vi "Begin.vi"(8 "error in":errorcluster) -> (0 "error out":errorcluster)   [LabVIEW 2015]
doc: "Called before other user functions, this VI is expected to open initial I/O refnums, load in file data, and do all program initialization. Notice that the <B>error out</B> terminal is simply used for data flow. Wiring it to other structures or subVIs ensures that this VI runs first."
uses:
  <vilib>/Rock Robotics/SystemInterfaces/i2clib/i2c_bus.ctl
  <vilib>/Rock Robotics/WPI/DriverStation/WPI_DriverStationRobotMode2.ctl
  <vilib>/Rock Robotics/SystemInterfaces/DIO/FPGA_DIOPWMChannel.ctl
  <vilib>/Rock Robotics/SystemInterfaces/spilib/spi_bus.ctl
  <vilib>/Rock Robotics/WPI/Accelerometer/WPI_AccelerometerADXL345 Axes.ctl
  <vilib>/Rock Robotics/WPI/Accelerometer/ADXL362 Range.ctl
  Robot Global Data.vi
  <vilib>/Rock Robotics/Network Tables/NT Write String Array.vi
  Team Code/Global_Var/Drive_Global.vi
  <vilib>/Rock Robotics/WPI/Gyro/WPI_GyroXRS450_SPI_Open.vi
  <vilib>/Rock Robotics/WPI/Accelerometer/WPI_AccelerometerADXL362_SPI_Open.vi
panel:
  in  "Comp_Robot?":bool=TRUE
  out "IMU Cal Result":T1={"AccelCalGood"=FALSE, "GyroCalGood"=TRUE, "MagCalGood"=FALSE, "Accel_StdDev"=0.2675184573071548, "Gyro_StdDev"=0.04462048242979951}
  in  "NumCalSamples":i32=50
  in  "Accel-Gyro_Settings":T2={"Accel_Range"=enum."±4g", "Gyro_Range"=enum."±500dps", "A/G_Address"=enum."0x6B", "Motion Thresh"=0.0, "reset"=FALSE}
  in  "Mag_Settings":T3={"Mag_Range"=enum."±2 gauss", "Mag_Address"=enum."0x1E", "Anomaly Thresh"=0.0, "Local Mag"=0.0}
  in  "I2C Bus":T4
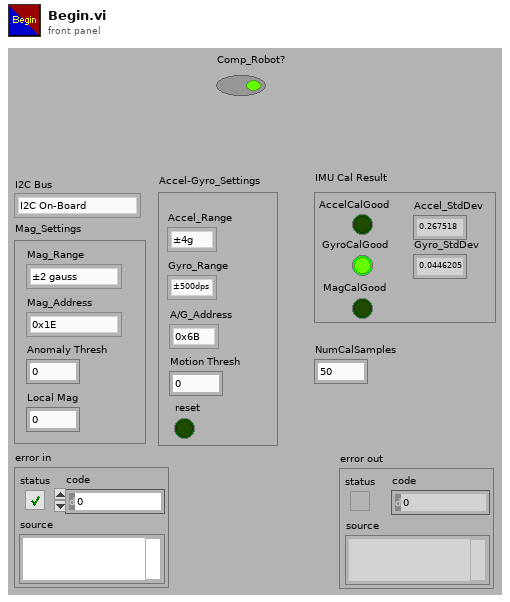
[diagram p1: front panel]
types:
  T1 = cluster{"AccelCalGood":bool, "GyroCalGood":bool, "MagCalGood":bool, "Accel_StdDev":dbl, "Gyro_StdDev":dbl}
  T2 = cluster{"Accel_Range":enum8{"±2g", "±16g", "±4g", "±8g", "disabled"}, "Gyro_Range":enum8{"±245dps", "±500dps", "disabled", "±2000dps"}, "A/G_Address":enum8{"0x6A", "0x6B"}, "Motion Thresh":dbl, "reset":bool}
  T3 = cluster{"Mag_Range":enum8{"±2 gauss", "±4 gauss", "±8 gauss", "±16 gauss", "disabled"}, "Mag_Address":enum8{"0x1C", "0x1E"}, "Anomaly Thresh":dbl, "Local Mag":dbl}
  T4 = typedef "i2c_bus.ctl" = enum16{"I2C On-Board", "I2C MXP", "Invalid"}
  T5 = typedef "ADXL362 Range.ctl" = u8
  T6 = typedef "WPI_AccelerometerADXL345 Axes.ctl" = cluster{"X-Axis":bool, "Y-Axis":bool, "Z-Axis":bool}
  T7 = typedef "spi_bus.ctl" = enum16{"SPI On-Board, CS0", "SPI On-Board, CS1", "SPI On-Board, CS2", "SPI On-Board, CS3", "SPI MXP", "Invalid"}
  T8 = typedef "FPGA_DIOPWMChannel.ctl" = enum8{"PWM 0", "PWM 1", "PWM 2", "PWM 3", "PWM 4", "PWM 5", "PWM 6", "PWM 7", "PWM 8", "PWM 9", "PWM MXP 0", "PWM MXP 1", "PWM MXP 2", "PWM MXP 3", "PWM MXP 4", "PWM MXP 5", "PWM MXP 6", "PWM MXP 7", "PWM MXP 8", "PWM MXP 9", "Invalid"}
  T9 = typedef "WPI_DriverStationRobotMode2.ctl" = enum16{"Autonomous Disabled", "Autonomous Enabled", "Teleop Disabled", "Teleop Enabled", "Disconnected", "Finish", "Test Disabled", "Test Enabled", "Emergency Stopped"}
  T10 = typedef "LSM9DS1DevRef.ctl" = cluster{"DevStatus":errorcluster, "Gyro Offset":cluster{"Xzero":dbl, "Yzero":dbl, "Zzero":dbl}, "StdDev Rates":cluster{"Xsdo":dbl, "Ysdo":dbl, "Zsdo":dbl}, "Reset":bool, "Accel Offset":cluster{"Xzero":dbl, "Yzero":dbl, "Zzero":dbl}, "Motion Thresh":dbl, "Mag Offset":cluster{"Xzero":dbl, "Yzero":dbl, "Zzero":dbl}, "I2C Bus":T4, "Handle":i32, "Anomaly Thresh":dbl, "Local Mag":dbl, "Accel/Gyro_Address":enum8{"0x6A", "0x6B"}, "Accel_Range":enum16{"±2g", "±16g", "±4g", "±8g", "disabled"}, "Gyro_Range":enum16{"±245dps", "±500dps", "disabled", "±2000dps"}, "Mag_Range":enum16{"±2 gauss", "±4 gauss", "±8 gauss", "±16 gauss", "disabled"}, "Mag_Address":enum8{"0x1C", "0x1E"}, "accel_active":bool, "gyro_active":bool, "mag_active":bool}
  T11 = typedef "WPI_ServoDeviceRef.ctl" = cluster{"DeviceStatus":errorcluster, "PWM Channel":T8, "DeadBand":T12}
  T12 = typedef "WPI_PWMDeadband.ctl" = cluster{"Name":string, "maxPositivePwm":i32, "minPositivePwm":i32, "centerPwm":i32, "maxNegativePwm":i32, "minNegativePwm":i32, "angularRange":u16}
  T13 = typedef "WPI_GyroDevRef.ctl" = cluster{"DevStatus":errorcluster, "Analog Channel":T14, "Offset":dbl, "Gain (VoltsPerDegree/Second)":dbl, "Gyro Type":enum16{"Analog", "XRS450"}, "Handle":i32, "SPI Bus":T7, "Device Found":bool, "Sample Rate":dbl, "Calibrate On Open":bool}
  T14 = typedef "FPGA_AIChannel.ctl" = enum8{"AI 0", "AI 1", "AI 2", "AI 3", "AI MXP 0", "AI MXP 1", "AI MXP 2", "AI MXP 3", "Invalid"}
  T15 = typedef "WPI_AccelerometerDevRef.ctl" = cluster{"DevStatus":errorcluster, "Scaling":T16, "Analog Channels":T17, "I2C Bus":T4, "SPI Bus":T7, "Accel Range":T18, "ADXL Axes":T6, "Handle":i32, "Device Address":u8, "Accel Type":enum16{"Analog", "ADXL345 I2C", "ADXL345 SPI", "Internal", "ADXL362 SPI"}}
  T16 = typedef "WPI_AccelerometerScaling.ctl" = cluster{"Gain (VoltsPerG)":dbl, "Center Voltage":dbl}
  T17 = typedef "WPI_AccelerometerAnalogChannels.ctl" = cluster{"X-Axis":T14, "Y-Axis":T14, "Z-Axis":T14}
  T18 = typedef "ADXL345 Range.ctl" = u8
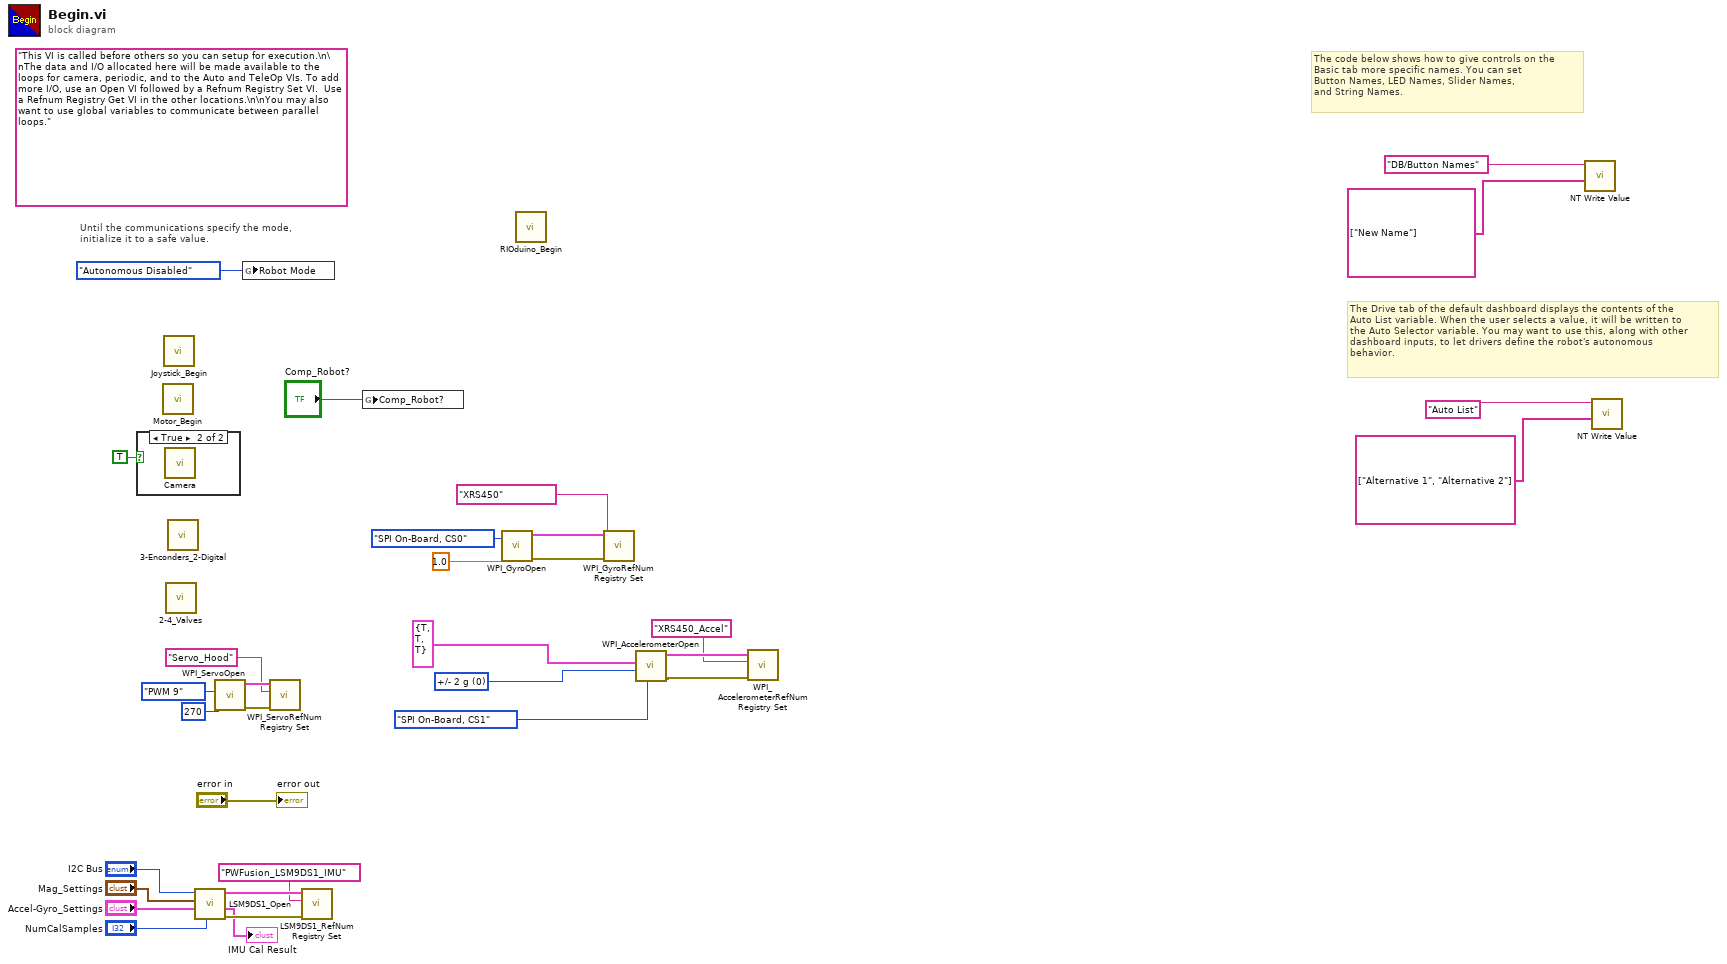
[diagram p0: block diagram]
diagram:
  w5 = T5 0 items=["+/- 2 g", "+/- 4 g", "+/- 8 g"] ("Accel Range")
  (unwired) "This VI is called before others so you can setup for execution.\n\nThe data and I/O allocated here will be made available to the loops for camera, periodic, and to the Auto and TeleOp VIs. To add more I/O, use an Open VI followed by a Refnum Registry Set VI.  Use a Refnum Registry Get VI in the other locations.\n\nYou may also want to use global variables to communicate between parallel loops."
  # "The Drive tab of the default dashboard displays the contents of the\nAuto List variable. When the user selects a value, it will be written to\nthe Auto Selector variable. You may want to use this, along with other\ndashboard inputs, to let drivers define the robot's autonomous\nbehavior."
  # "The code below shows how to give controls on the\nBasic tab more specific names. You can set\nButton Names, LED Names, Slider Names,\nand String Names."
  # "Until the communications specify the mode,\ninitialize it to a safe value."
  n1 = case shown="True" TRUE {
    frame False {
    }
    frame True {
      n2 = call "Camera.vi"() -> ()  [unwired: 12 in]
    }
  }
  n3 = call "Motor_Begin.vi"() -> ()  [unwired: 12 in]
  n4 = call "Joystick_Begin.vi"() -> ()  [unwired: 12 in]
  n5 = call "2-4_Valves.vi"() -> ()  [unwired: 12 in]
  n6 = call "3-Enconders_2-Digital.vi"() -> ()  [unwired: 12 in]
  n7 = call "LSM9DS1_Open.vi"("NumCalSamples"="NumCalSamples", "Accel-Gyro_Settings"="Accel-Gyro_Settings", "Mag_Settings"="Mag_Settings", "I2C Bus"="I2C Bus") -> ("error out"=w23:errorcluster, "IMU Cal Result"=→"IMU Cal Result":T1, "LSM9DS1DevRef Out"=w25:T10)  [unwired: 5 in]
  n8 = call <vilib>:"WPI_ServoOpen.vi"("Angular Range"=u16 270, "PWM Channel"=FPGA_DIOPWMChannel."PWM 9") -> ("error out"=w16:errorcluster, "ServoDeviceRef"=w15:T11)  [unwired: 8 in]
  n9 = global write "Robot Global Data.vi" "Robot Mode"(WPI_DriverStationRobotMode2."Autonomous Disabled" ("Robot Mode")) -> ()
  n10 = call <vilib>:"WPI_ServoRefNum Registry Set.vi"("error in (no error)"=w16, "refnum name"="Servo_Hood", "ServoDeviceRef"=w15) -> ()  [unwired: 7 in, 2 out]
  n11 = call "LSM9DS1_RefNum Registry Set.vi"("error in (no error)"=w23, "refnum name"="PWFusion_LSM9DS1_IMU", "LSM9DS1DevRef"=w25) -> ()  [unwired: 7 in, 2 out]
  n12 = global write "Drive_Global.vi" "Comp_Robot?"("Comp_Robot?") -> ()
  n13 = call-poly <vilib>:"WPI_GyroOpen.vi"("Sample Rate (ms)"=1.0, "SPI Bus"=spi_bus."SPI On-Board, CS0") -> ("error out"=w9:errorcluster, "GyroDevRef"=w10:T13)  [unwired: 8 in]
  n14 = call "RIOduino_Begin.vi"() -> ()  [unwired: 12 in]
  n15 = call <vilib>:"WPI_GyroRefNum Registry Set.vi"("error in (no error)"=w9, "refnum name"="XRS450", "GyroDevRef"=w10) -> ()  [unwired: 7 in, 2 out]
  n16 = call-poly <vilib>:"WPI_AccelerometerOpen.vi"("SPI Bus"=spi_bus."SPI On-Board, CS1", "Accel Range"=w5, "ADXL345 Axes"=T6 {"X-Axis"=TRUE, "Y-Axis"=TRUE, "Z-Axis"=TRUE}) -> ("error out"=w3:errorcluster, "AccelerometerDevRef"=w4:T15)  [unwired: 7 in]
  n17 = call <vilib>:"WPI_AccelerometerRefNum Registry Set.vi"("error in (no error)"=w3, "refnum name"="XRS450_Accel", "AccelerometerDevRef"=w4) -> ()  [unwired: 7 in, 2 out]
  n18 = call-poly <vilib>:"NT Write Value.vi"("String Array"=string[] ["New Name"], "Name"="DB/Button Names") -> ()  [unwired: 9 in, 1 out]
  n19 = call-poly <vilib>:"NT Write Value.vi"("String Array"=string[] ["Alternative 1", "Alternative 2"], "Name"="Auto List") -> ()  [unwired: 9 in, 1 out]
  "error out" <- "error in"
